vi "Write.vi"(8 "error in (no error)":errorcluster, 11 "CSV_Writer in":refnum<class "CSV_Writer.lvclass">) -> (0 "error out":errorcluster, 3 "CSV_Writer out":refnum<class "CSV_Writer.lvclass">)   [LabVIEW 2024, in "Data.lvlib" / "CSV_Writer.lvclass"]
uses:
  CSV_Writer.lvclass
  CSV_Writer.lvclass/CSV_Writer.ctl
  Data/DataWriter/DataWriter.lvclass
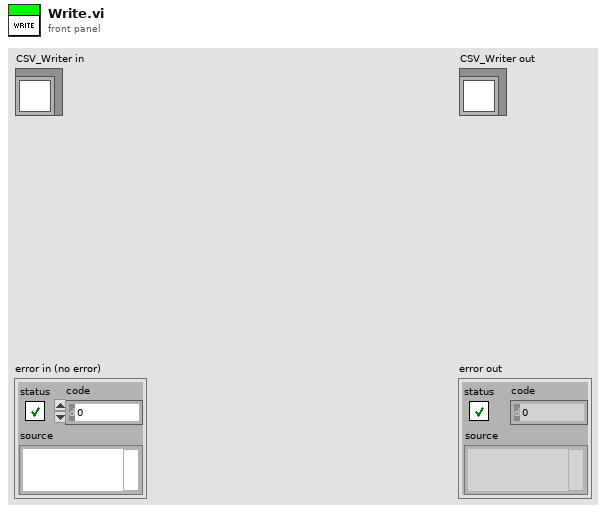
[diagram p1: front panel]
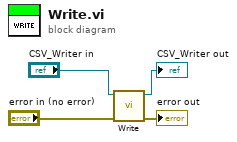
[diagram p0: block diagram]
diagram:
  n1 = call-parent "Write.vi"("error in (no error)"="error in (no error)", "DataWriter in"="CSV_Writer in") -> ("error out"=→"error out":errorcluster, "DataWriter out"=→"CSV_Writer out":refnum<class "CSV_Writer.lvclass">)  [unwired: 8 in]
